vi "FRCts20_WebMethods_Single_Request_GET.vi"(7 "LabVIEW Web Service Request":refnum<class "Web Request.lvclass">, 10 "ReqNumber":string="-1") -> ()   [LabVIEW 2014, in "FRCts20_WebMethods.lvlib"]
doc: "<B>GET</B> on the specified <B>request</B> resource\n\nIf request is not specified, will return all resources. Requests can be filtered using the following parameters in the query string:\n - <B>division</B>\n - <B>team</B>\n - <B>status</B> (Open, In Work, Closed)\n\nhttp://<server address>:<port>/FRCts/request/<B>request</B>"
uses:
  FRCts20_WebMethods.lvlib
  <vilib>/wsapi/Web Request.lvclass
  Backend/source/VI Source/FRCts20_Backend_API/Requests.ctl
  Backend/source/VI Source/FRCts20_Backend_API/Request.ctl
  Backend/source/VI Source/FRCts20_Backend_API/ApiReturn.ctl
  Backend/source/VI Source/FRCts20_Backend_API/FRCts20_Backend_API_Status.ctl
  Backend/source/VI Source/FRCts20_Backend_API/NotesRoot.ctl
  Backend/source/VI Source/FRCts20_Backend_API/FRCts20_Backend_API_Command_Request.ctl
  Backend/source/VI Source/FRCts20_Backend_API/FRCts20_Backend_API_Request.vi
  Backend/source/VI Source/FRCts20_Backend_API/FRCts20_Backend_API.lvlib
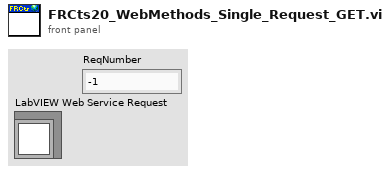
[diagram p1: front panel]
types:
  T1 = typedef "FRCts20_Backend_Engine.lvlib/FRCts20_Backend_API.lvlib/Request.ctl" = cluster{"APIReturn":T2, "RequestRoot":cluster{"ReqNumber":i32, "Description":string, "Status":T3, "Open Date":string, "Last Update":string, "Closed Date":string, "TeamIndex":i32, "EventIndex":i32}, "Notes":T4}
  T2 = typedef "FRCts20_Backend_Engine.lvlib/FRCts20_Backend_API.lvlib/ApiReturn.ctl" = string
  T3 = typedef "FRCts20_Backend_Engine.lvlib/FRCts20_Backend_API.lvlib/FRCts20_Backend_API_Status.ctl" = i32
  T4 = typedef "FRCts20_Backend_Engine.lvlib/FRCts20_Backend_API.lvlib/NotesRoot.ctl" = cluster{"NoteIndex":u32, "ReqNumber":i32, "NoteText":string, "TimeEntered":string, "Author":string, "Solution":bool, "Deleted":bool}[]
  T5 = typedef "FRCts20_Backend_Engine.lvlib/FRCts20_Backend_API.lvlib/FRCts20_Backend_API_Command_Request.ctl" = string
  T6 = typedef "FRCts20_Backend_Engine.lvlib/FRCts20_Backend_API.lvlib/Requests.ctl" = cluster{"APIReturn":string, "Request Array":T1[]}
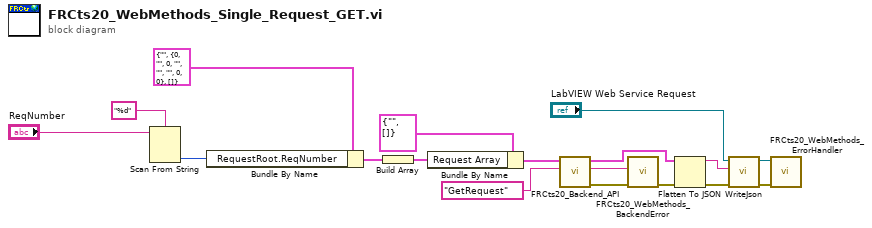
[diagram p0: block diagram]
diagram:
  n1 = Scan From String(format string="%d", input string="ReqNumber") -> (output 1=w1:i32)  [unwired: 3 in, 3 out]
  n2 = Bundle By Name(cluster=T1 {"APIReturn"="", "RequestRoot"={"ReqNumber"=0, "Description"="", "Status"=0, "Open Date"="", "Last Update"="", "Closed Date"="", "TeamIndex"=0, "EventIndex"=0}, "Notes"=[]} ("Request"), "RequestRoot.ReqNumber"=w1) -> (w12:T1)
  n3 = Build Array(w12) -> (w11:T1[])
  n4 = Bundle By Name(cluster=T6 {"APIReturn"="", "Request Array"=[]} ("Requests"), "Request Array"=w11) -> (w10:T6)
  n5 = call-poly "FRCts20_Backend_API.vi"("Command"=T5 "GetRequest", "Request In"=w10) -> ("error out"=w17:errorcluster, "Status"=w18:string, "Request Out"=w4:T6)  [unwired: 7 in]
  n6 = call "FRCts20_WebMethods_BackendError.vi"("error in (no error)"=w17, "Status"=w18) -> ("error out"=w16:errorcluster)  [unwired: 8 in, 1 out]
  n7 = Flatten To JSON(anything=w4, error in (no error)=w16) -> (JSON string=w5:string, 11:w9:errorcluster)  [unwired: 1 in]
  n8 = call "WriteJson.vi"("error in (no error)"=w9, "JSON string"=w5, "Web Request in"="LabVIEW Web Service Request") -> ("error out"=w8:errorcluster, "Web Request out"=w6:refnum<class "Web Request.lvclass">)  [unwired: 7 in]
  n9 = call "FRCts20_WebMethods_ErrorHandler.vi"("error in"=w8, "LabVIEW Web Service Request"=w6) -> ()  [unwired: 8 in, 2 out]
